vi "test Add RAF Channel.vi"(8 "error in (no error)":errorcluster, 11 "TestCase in":refnum<class "Routing and Faulting Scripting Unit Tests.lvclass">) -> (0 "error out":errorcluster, 3 "TestCase out":refnum<class "Routing and Faulting Scripting Unit Tests.lvclass">)   [LabVIEW 2020, in "Routing and Faulting Scripting Unit Tests.lvclass"]
uses:
  Routing and Faulting Scripting Unit Tests.lvclass
  Shared/Channel States.ctl
  Shared/Routing State.ctl
  Shared/Connection.ctl
  Routing and Faulting Scripting Unit Tests.lvclass/Routing and Faulting Scripting Unit Tests.ctl
  <vilib>/addons/_JKI Toolkits/VI Tester/TestCase.llb/TestCase.lvclass
  Routing and Faulting Scripting.lvlib
  Shared/Routing and Faulting Shared.lvlib
  C:/Program Files (x86)/National Instruments/LabVIEW 2020/vi.lib/addons/_JKI Toolkits/VI Tester/TestCase.llb/TestCase.lvclass
panel:
  in  "Save?":bool
  out "Output Filename":string
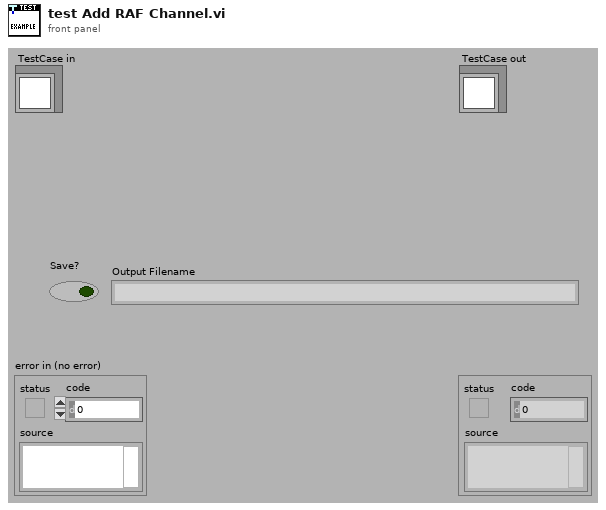
[diagram p1: front panel]
types:
  T1 = typedef "Routing and Faulting Shared.lvlib/Channel States.ctl" = T2[]
  T2 = typedef "Routing and Faulting Shared.lvlib/Routing State.ctl" = cluster{"Name":string, "Description":string, "Value":i32, "Connection List":T3[]}
  T3 = typedef "Routing and Faulting Shared.lvlib/Connection.ctl" = cluster{"Module":string, "Source":string, "Destination":string}
  T4 = typedef "Custom Device API.lvlib/Custom Device Item Ref.ctl" = u64
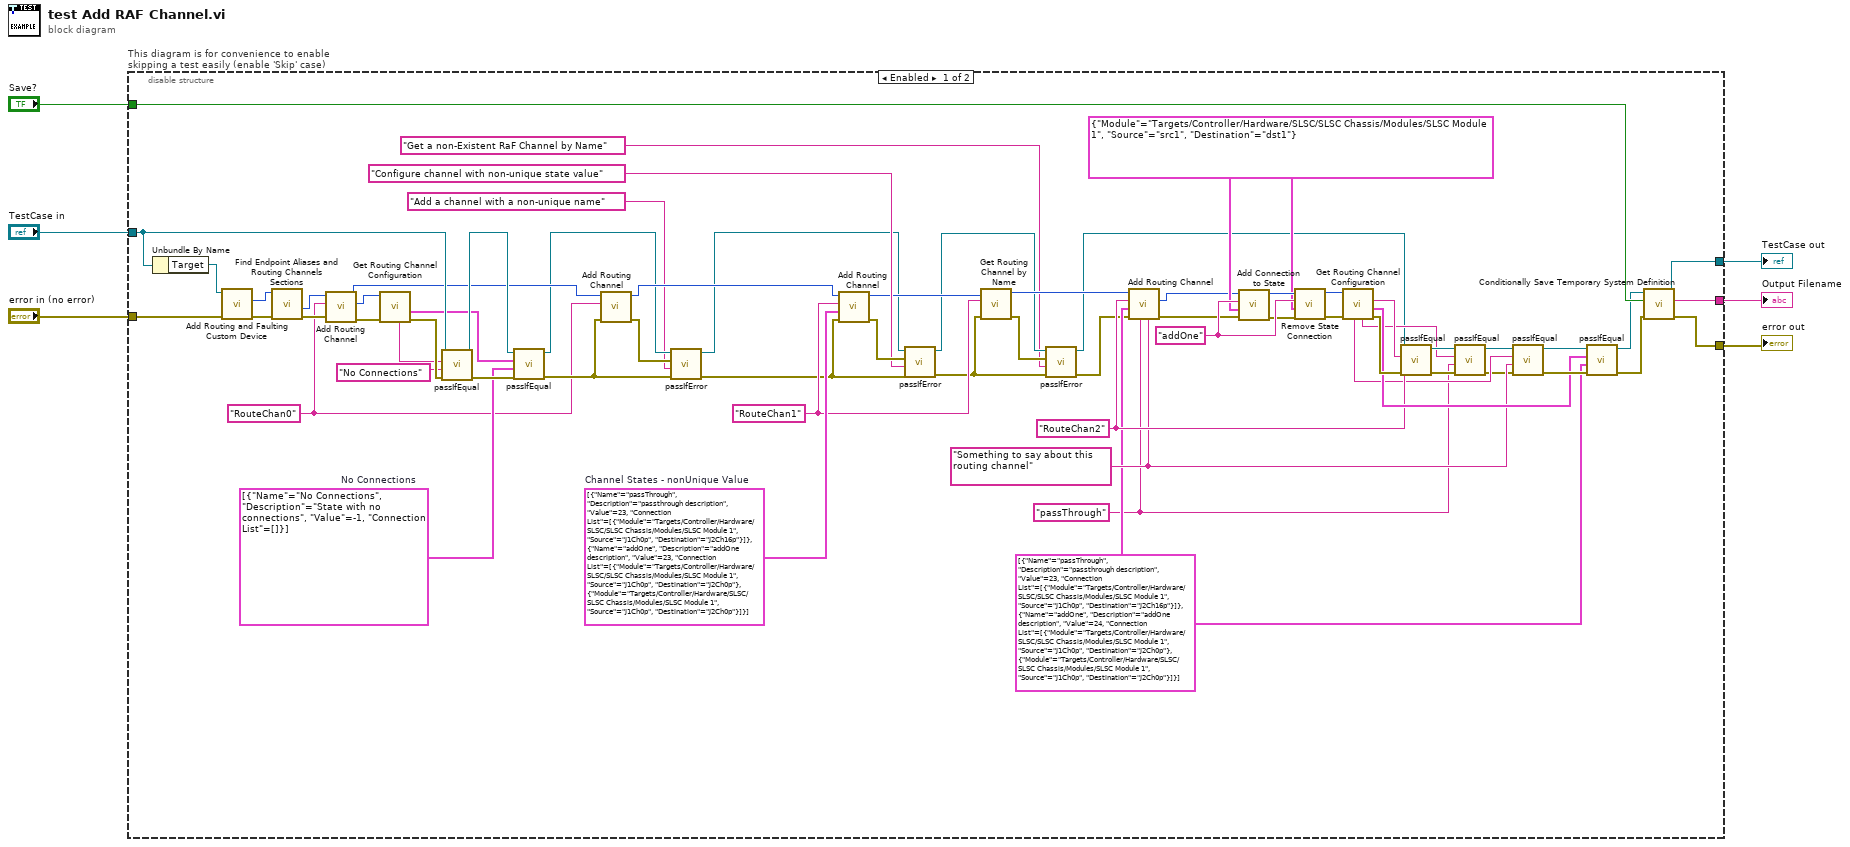
[diagram p0: block diagram]
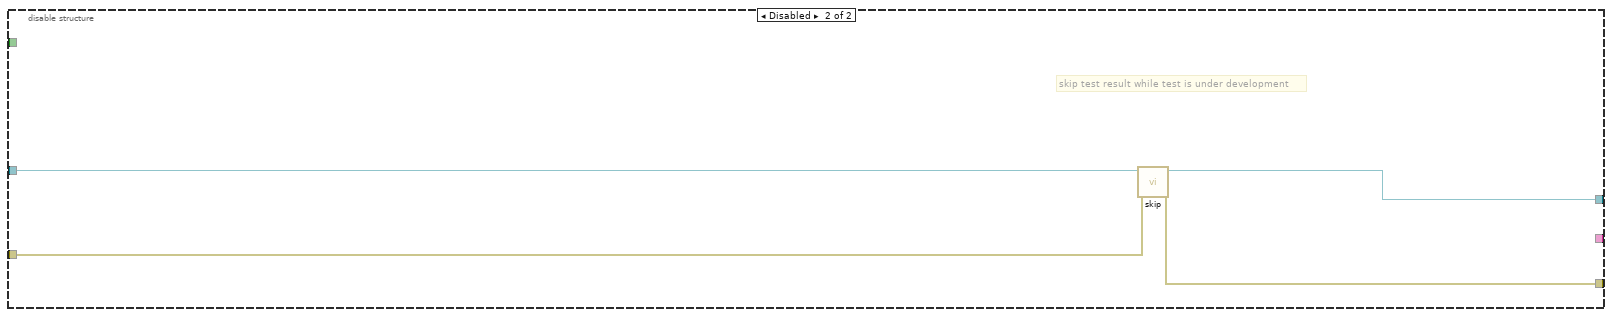
[diagram p2: hidden frame]
diagram:
  n1 = disable-structure "This diagram is for convenience to enable skipping a test easily (enable 'Skip' case)" shown="Enabled" {
    disable-tunnel: "TestCase in" -> [w32 w76]
    disable-tunnel: [w67 w74] -> w3
    disable-tunnel: [w71 w75] -> w5
    disable-tunnel: "error in (no error)" -> [w72 w73]
    disable-tunnel: [w70 _] -> w2
    disable-tunnel: "Save?" -> [w69 _]
    frame Enabled {
      w25 = T1 [{"Name"="No Connections", "Description"="State with no connections", "Value"=-1, "Connection List"=[]}]  # No Connections
      w8 = "RouteChan0" ("Channel Name")
      w36 = "passThrough" ("Name")
      w24 = "RouteChan1" ("Channel Name")
      w46 = T1 [{"Name"="passThrough", "Description"="passthrough description", "Value"=23, "Connection List"=[{"Module"="Targets/Controller/Hardware/SLSC/SLSC Chassis/Modules/SLSC Module 1", "Source"="J1Ch0p", "Destination"="J2Ch16p"}]}, {"Name"="addOne", "Description"="addOne description", "Value"=23, "Connection List"=[{"Module"="Targets/Controller/Hardware/SLSC/SLSC Chassis/Modules/SLSC Module 1", "Source"="J1Ch0p", "Destination"="J2Ch0p"}, {"Module"="Targets/Controller/Hardware/SLSC/SLSC Chassis/Modules/SLSC Module 1", "Source"="J1Ch0p", "Destination"="J2Ch0p"}]}]  # Channel States - nonUnique Value
      w48 = "Something to say about this routing channel" ("Description")
      w61 = T3 {"Module"="Targets/Controller/Hardware/SLSC/SLSC Chassis/Modules/SLSC Module 1", "Source"="src1", "Destination"="dst1"} ("connection")
      w62 = "addOne" ("state name")
      w42 = T1 [{"Name"="passThrough", "Description"="passthrough description", "Value"=23, "Connection List"=[{"Module"="Targets/Controller/Hardware/SLSC/SLSC Chassis/Modules/SLSC Module 1", "Source"="J1Ch0p", "Destination"="J2Ch16p"}]}, {"Name"="addOne", "Description"="addOne description", "Value"=24, "Connection List"=[{"Module"="Targets/Controller/Hardware/SLSC/SLSC Chassis/Modules/SLSC Module 1", "Source"="J1Ch0p", "Destination"="J2Ch0p"}, {"Module"="Targets/Controller/Hardware/SLSC/SLSC Chassis/Modules/SLSC Module 1", "Source"="J1Ch0p", "Destination"="J2Ch0p"}]}] ("Channel States")
      w51 = "RouteChan2" ("Channel Name")
      n2 = Unbundle By Name(w32) -> ("Target"=w68:refnum<k24>)
      n3 = call "Add Routing and Faulting Custom Device.vi"("error in"=w72, "target in"=w68) -> ("error out"=w66:errorcluster, "routing and faulting custom device"=w49:T4)  [unwired: 7 in, 1 out]
      n4 = call "Find Endpoint Aliases and Routing Channels Sections.vi"("error in"=w66, "routing and faulting custom device in"=w49) -> ("error out"=w44:errorcluster, "routing channels"=w34:T4)  [unwired: 6 in, 2 out]
      n5 = call "Add Routing Channel.vi"("error in"=w44, "channel name"=w8, "routing channels in"=w34) -> ("error out"=w35:errorcluster, "routing channel"=w29:T4, "routing channels out"=w15:T4)  [unwired: 6 in]
      n6 = call "Get Routing Channel Configuration.vi"("error in"=w35, "routing channel in"=w29) -> ("error out"=w33:errorcluster, "state configurations"=w26:T1, "initial state"=w31:string)  [unwired: 4 in, 3 out]
      n7 = call-dynamic "passIfEqual.vi"("error in (no error)"=w33, "y"="No Connections" ("Initial State"), "x"=w31, "TestCase in"=w32) -> ("error out"=w28:errorcluster, "TestCase out"=w27:refnum<class "Routing and Faulting Scripting Unit Tests.lvclass">)  [unwired: 6 in]
      n8 = call-dynamic "passIfEqual.vi"("error in (no error)"=w28, "y"=w25, "x"=w26, "TestCase in"=w27) -> ("error out"=w12:errorcluster, "TestCase out"=w10:refnum<class "Routing and Faulting Scripting Unit Tests.lvclass">)  [unwired: 6 in]
      n9 = call "Add Routing Channel.vi"("error in"=w12, "channel name"=w8, "routing channels in"=w15) -> ("error out"=w13:errorcluster, "routing channels out"=w14:T4)  [unwired: 6 in, 1 out]
      n10 = call-dynamic "passIfError.vi"("error in (no error)"=w12, "task (\"\")"="Add a channel with a non-unique name" ("task (\"\")"), "error"=w13, "TestCase in"=w10) -> ("error out"=w11:errorcluster, "TestCase out"=w9:refnum<class "Routing and Faulting Scripting Unit Tests.lvclass">)  [unwired: 6 in]
      n11 = call "Add Routing Channel.vi"("error in"=w11, "state configurations"=w46, "channel name"=w24, "routing channels in"=w14) -> ("error out"=w45:errorcluster, "routing channels out"=w23:T4)  [unwired: 5 in, 1 out]
      n12 = call-dynamic "passIfError.vi"("error in (no error)"=w11, "task (\"\")"="Configure channel with non-unique state value" ("task (\"\")"), "error"=w45, "TestCase in"=w9) -> ("error out"=w18:errorcluster, "TestCase out"=w20:refnum<class "Routing and Faulting Scripting Unit Tests.lvclass">)  [unwired: 6 in]
      n13 = call "Get Routing Channel by Name.vi"("error in"=w18, "channel name"=w24, "routing channels in"=w23) -> ("error out"=w17:errorcluster, "routing channels out"=w22:T4)  [unwired: 6 in, 1 out]
      n14 = call-dynamic "passIfError.vi"("error in (no error)"=w18, "task (\"\")"="Get a non-Existent RaF Channel by Name" ("task (\"\")"), "error"=w17, "TestCase in"=w20) -> ("error out"=w21:errorcluster, "TestCase out"=w19:refnum<class "Routing and Faulting Scripting Unit Tests.lvclass">)  [unwired: 6 in]
      n15 = call "Add Routing Channel.vi"("description"=w48, "initial state"=w36, "error in"=w21, "state configurations"=w42, "channel name"=w51, "routing channels in"=w22) -> ("error out"=w58:errorcluster, "routing channel"=w56:T4)  [unwired: 3 in, 1 out]
      n16 = call "Add Connection to State.vi"("error in"=w58, "connection"=w61, "state"=w62, "routing channel in"=w56) -> ("error out"=w59:errorcluster, "routing channel out"=w63:T4)  [unwired: 6 in]
      n17 = call "Remove State Connection.vi"("error in"=w59, "connection"=w61, "state"=w62, "routing channel in"=w63) -> ("error out"=w60:errorcluster, "routing channel out"=w57:T4)  [unwired: 6 in]
      n18 = call "Get Routing Channel Configuration.vi"("error in"=w60, "routing channel in"=w57) -> ("error out"=w54:errorcluster, "state configurations"=w52:T1, "routing channel name"=w50:string, "initial state"=w37:string, "description"=w47:string)  [unwired: 4 in, 1 out]
      n19 = call-dynamic "passIfEqual.vi"("error in (no error)"=w54, "y"=w51, "x"=w50, "TestCase in"=w19) -> ("error out"=w41:errorcluster, "TestCase out"=w38:refnum<class "Routing and Faulting Scripting Unit Tests.lvclass">)  [unwired: 6 in]
      n20 = call-dynamic "passIfEqual.vi"("error in (no error)"=w41, "y"=w36, "x"=w37, "TestCase in"=w38) -> ("error out"=w40:errorcluster, "TestCase out"=w39:refnum<class "Routing and Faulting Scripting Unit Tests.lvclass">)  [unwired: 6 in]
      n21 = call-dynamic "passIfEqual.vi"("error in (no error)"=w40, "y"=w48, "x"=w47, "TestCase in"=w39) -> ("error out"=w53:errorcluster, "TestCase out"=w55:refnum<class "Routing and Faulting Scripting Unit Tests.lvclass">)  [unwired: 6 in]
      n22 = call-dynamic "passIfEqual.vi"("error in (no error)"=w53, "y"=w42, "x"=w52, "TestCase in"=w55) -> ("error out"=w65:errorcluster, "TestCase out"=w64:refnum<class "Routing and Faulting Scripting Unit Tests.lvclass">)  [unwired: 6 in]
      n23 = call "Conditionally Save Temporary System Definition.vi"("error in (no error)"=w65, "Save?"=w69, "Test Case"=w64) -> ("error out"=w71:errorcluster, "filename"=w70:string, "Test Case"=w67:refnum<class "Routing and Faulting Scripting Unit Tests.lvclass">)  [unwired: 6 in]
    }
    frame Disabled {
      # "skip test result while test is under development"
      n24 = call <vilib>:"skip.vi"("error in (no error)"=w73, "TestCase in"=w76) -> ("error out"=w75:errorcluster, "TestCase out"=w74:refnum<class "Routing and Faulting Scripting Unit Tests.lvclass">)  [unwired: 8 in]
    }
  }
  "error out" <- w5
  "TestCase out" <- w3
  "Output Filename" <- w2
